vi "AlliGator Load Single Gate Image from Piccolo hist .bin File.vi"(6 "Action":T1, 8 "error in (no error)":errorcluster, 10 "File Info":variant, 11 "Gate Index":i32) -> (0 "error out":errorcluster, 1 "Data 2":sgl[][](array[numeric]), 3 "Data 1":sgl[][](array[numeric]))   [LabVIEW 2021, in "AlliGator Files.lvlib"]
doc: "Single gate image loading step for Piccolo .bin files."
uses:
  AlliGator Files.lvlib
  HDF5/AlliGator FLI Image Stack Action.ctl
  AlliGator Piccolo hist .bin Dataset Information.ctl
  AlliGator Piccolo hist BIN File Information.ctl
  HDF5/AlliGator HDF5.lvlib
panel:
  # "see the AlliGator License on the block diagram (Ctrl+E or Window:Show Block Diagram)"
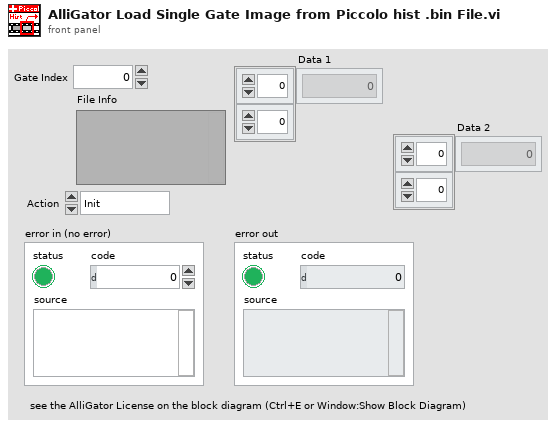
[diagram p1: front panel]
types:
  T1 = typedef "AlliGator HDF5.lvlib/AlliGator FLI Image Stack Action.ctl" = enum16{"Init", "Get Image", "Close"}
  T2 = typedef "AlliGator Files.lvlib/AlliGator Piccolo hist .bin Dataset Information.ctl" = cluster{"File Path":path, "Piccolo hist BIN dataset Information":T3}
  T3 = typedef "AlliGator Files.lvlib/AlliGator Piccolo hist BIN File Information.ctl" = cluster{"# Pixels X":i32, "# Pixels Y":i32, "# TCSPC Bins":i32, "Temporal Resolution":dbl[unit]}
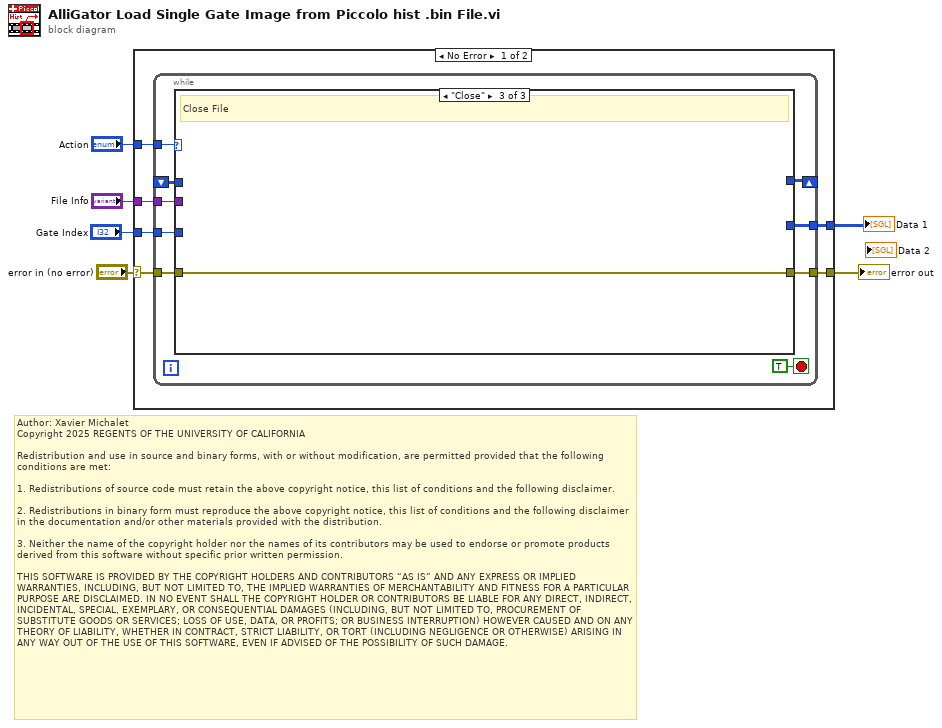
[diagram p0: block diagram]
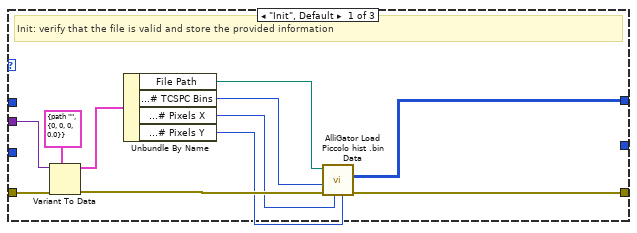
[diagram p2: hidden frame]
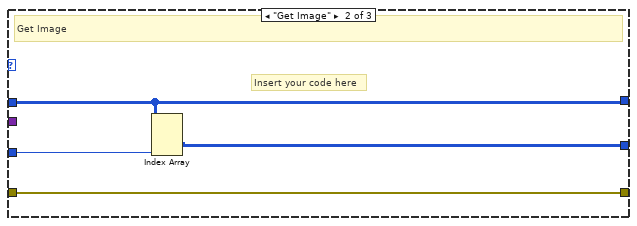
[diagram p3: hidden frame]
diagram:
  # "Author: Xavier Michalet\nCopyright 2025 REGENTS OF THE UNIVERSITY OF CALIFORNIA\n\nRedistribution and use in source and binary forms, with or without modification, are permitted provided that the following conditions are met:\n\n1. Redistributions of source code must retain the above copyright notice, this list of conditions and the following disclaimer.\n\n2. Redistributions in binary form must reproduce the above copyright notice, this list of conditions and the following disclaimer in the documentation and/or other materials provided with the distribution.\n\n3. Neither the name of the copyright holder nor the names of its contributors may be used to endorse or promote products derived from this software without specific prior written permission.\n\nTHIS SOFTWARE IS PROVIDED BY THE COPYRIGHT HOLDERS AND CONTRIBUTORS “AS IS” AND ANY EXPRESS OR IMPLIED WARRANTIES, INCLUDING, BUT NOT LIMITED TO, THE IMPLIED WARRANTIES OF MERCHANTABILITY AND FITNESS FOR A PARTICULAR PURPOSE ARE DISCLAIMED. IN NO EVENT SHALL THE COPYRIGHT HOLDER OR CONTRIBUTORS BE LIABLE FOR ANY DIRECT, INDIRECT, INCIDENTAL, SPECIAL, EXEMPLARY, OR CONSEQUENTIAL DAMAGES (INCLUDING, BUT NOT LIMITED TO, PROCUREMENT OF SUBSTITUTE GOODS OR SERVICES; LOSS OF USE, DATA, OR PROFITS; OR BUSINESS INTERRUPTION) HOWEVER CAUSED AND ON ANY THEORY OF LIABILITY, WHETHER IN CONTRACT, STRICT LIABILITY, OR TORT (INCLUDING NEGLIGENCE OR OTHERWISE) ARISING IN ANY WAY OUT OF THE USE OF THIS SOFTWARE, EVEN IF ADVISED OF THE POSSIBILITY OF SUCH DAMAGE."
  n1 = case shown="No Error" "error in (no error)" {
    selector: "error in (no error)" -> [w11 w38]
    tunnel: [w10 w38] -> w5
    tunnel: "Action" -> [w12 _]
    tunnel: "File Info" -> [w9 _]
    tunnel: "Gate Index" -> [w8 _]
    tunnel: [w7 _] -> w1
    frame No Error {
      n2 = while {
        tunnel: w12 -> [w20]
        tunnel: w11 -> [w19]
        tunnel: [w18] -> w10
        tunnel: w9 -> [w17]
        tunnel: w8 -> [w16]
        tunnel: [w15] -> w7
        shift-right: [w14] -> _
        shift-left: _ -> [w13]
        stop <- TRUE stop-if-true
        n3 = case shown="\"Close\"" w20 {
          tunnel: w19 -> [w31 w36 w37]
          tunnel: [w29 w36 w37] -> w18
          tunnel: w17 -> [w32 _ _]
          tunnel: w16 -> [_ w34 _]
          tunnel: [_ w33 _] -> w15
          tunnel: [w28 w35 _] -> w14
          tunnel: w13 -> [_ w35 _]
          frame "Init", Default {
            # "Init: verify that the file is valid and store the provided information"
            n4 = Variant To Data(error in=w31, type=T2 {"File Path"=path "", "Piccolo hist BIN dataset Information"={"# Pixels X"=0, "# Pixels Y"=0, "# TCSPC Bins"=0, "Temporal Resolution"=0.0}} ("Piccolo hist BIN Dataset Information"), Variant=w32) -> (data=w26:T2, error out=w30:errorcluster)
            n5 = Unbundle By Name(w26) -> ("File Path"=w25:path, "Piccolo hist BIN dataset Information.# TCSPC Bins"=w24:i32, "Piccolo hist BIN dataset Information.# Pixels X"=w23:i32, "Piccolo hist BIN dataset Information.# Pixels Y"=w22:i32)
            n6 = call "AlliGator Load Piccolo hist .bin Data.vi"("# Pixels Y"=w22, "# Pixels X"=w23, "error in (no error)"=w30, "# TCSPC Bins"=w24, "path in"=w25) -> ("error out"=w29:errorcluster, "Array"=w28:u16[][][])  [unwired: 4 in, 1 out]
          }
          frame "Get Image" {
            # "Insert your code here"
            # "Get Image"
            n7 = Index Array(array=w35, index (dim 2)=w34) -> (element=w33:u16[][])  [unwired: 2 in]
          }
          frame "Close" {
            # "Close File"
          }
        }
      }
    }
    frame Error {
    }
  }
  "Data 1" <- w1
  "error out" <- w5
